vi "Analysis.Result Summaries, Calculate Yield Metrics.vi"(5 "Total Cnt":i32, 6 "Retries":i32[](array[numeric]), 7 "Pass Cnt":i32, 8 "LP Fail":i32, 9 "LP Pass":i32, 10 "FP Fail":i32, 11 "FP Pass":i32) -> (3 "Metrics Table":string[][](table))   [LabVIEW 2024]
uses:
  Analysis.Yield Metrics.ctl
panel:
  out "Yield Metrics":T1 {"Retest"."Retested SN %" format="%.2f"; "Last Pass"."Yield%" format="%.2f"; "First Pass"."Yield%" format="%.2f"; "Overall"."Churn %" format="%.2f"; "Overall"."Yield%" format="%.2f"}
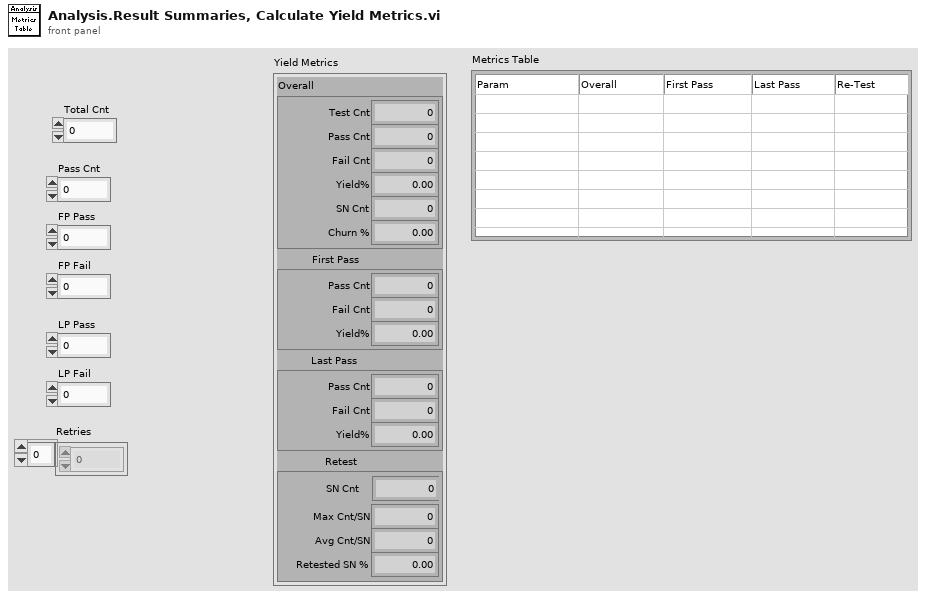
[diagram p1: front panel]
types:
  T1 = typedef "Analysis.Yield Metrics.ctl" = cluster{"Overall":cluster{"Pass Cnt":i32, "Fail Cnt":i32, "Yield%":dbl, "Test Cnt":i32, "SN Cnt":i32, "Churn %":dbl}, "First Pass":cluster{"Pass Cnt":i32, "Fail Cnt":i32, "Yield%":dbl}, "Last Pass":cluster{"Pass Cnt":i32, "Fail Cnt":i32, "Yield%":dbl}, "Retest":cluster{"Max Cnt/SN":i32, "Avg Cnt/SN":i32, "Retested SN %":dbl, "SN Cnt":i32}}
  T2 = cluster{"Pass Cnt":i32, "Fail Cnt":i32, "Yield%":dbl, "Test Cnt":i32, "SN Cnt":i32, "Churn %":dbl}
  T3 = cluster{"Max Cnt/SN":i32, "Avg Cnt/SN":i32, "Retested SN %":dbl, "SN Cnt":i32}
  T4 = cluster{"Pass Cnt":i32, "Fail Cnt":i32, "Yield%":dbl}
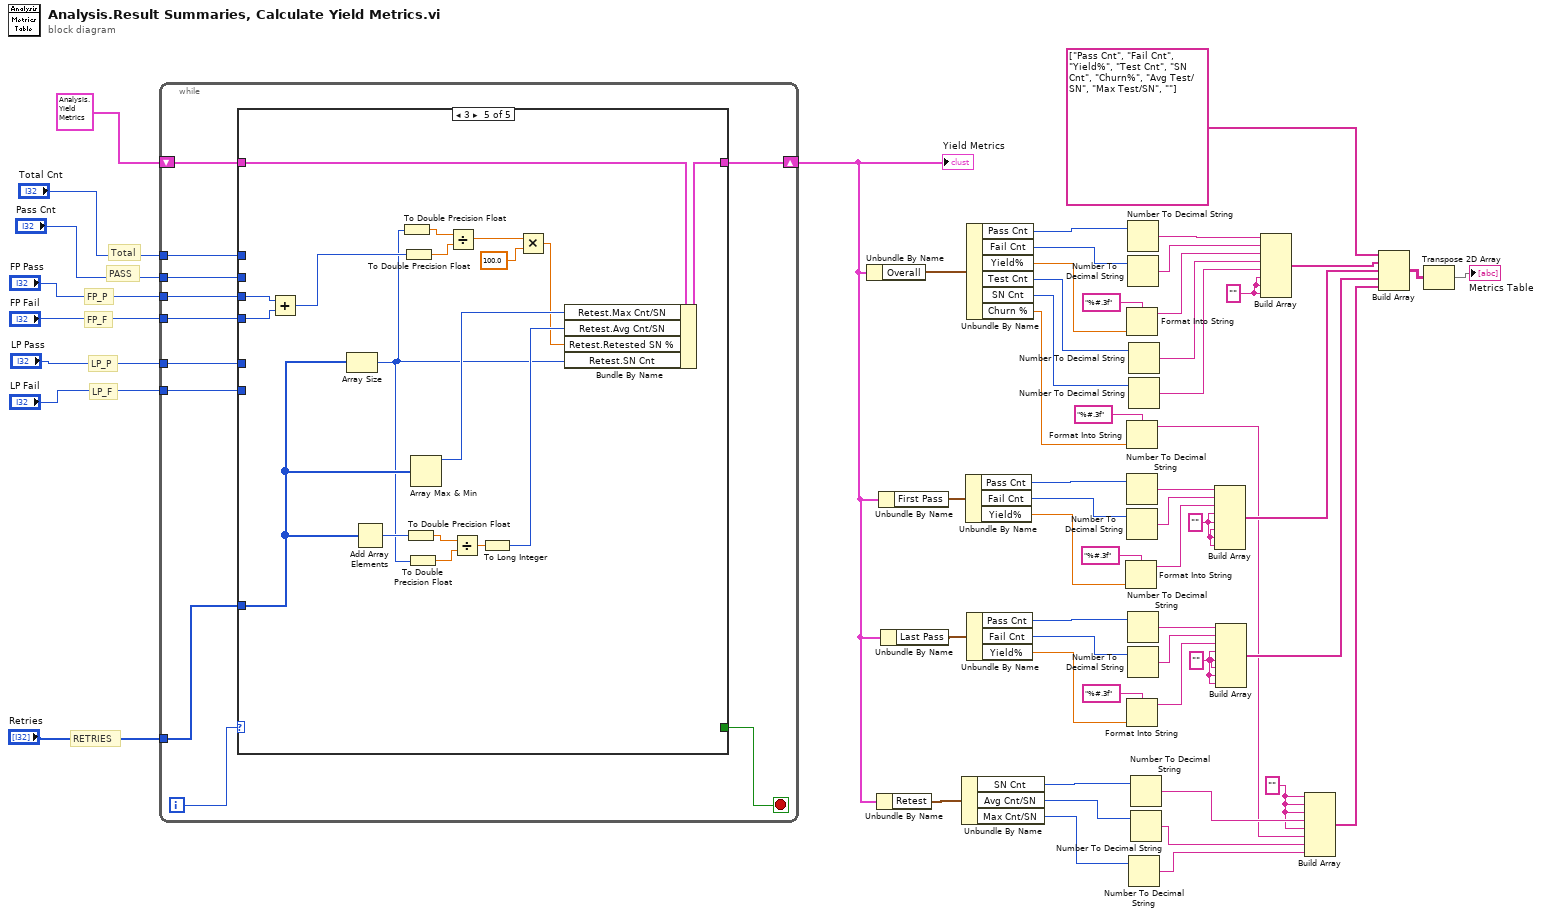
[diagram p0: block diagram]
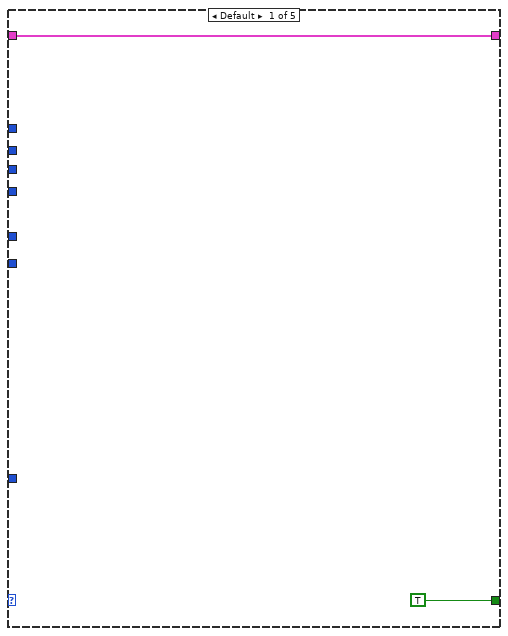
[diagram p2: hidden frame]
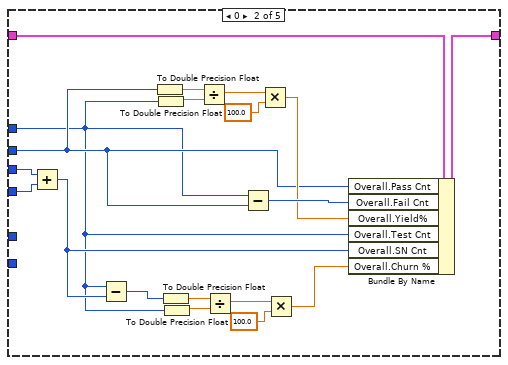
[diagram p3: hidden frame]
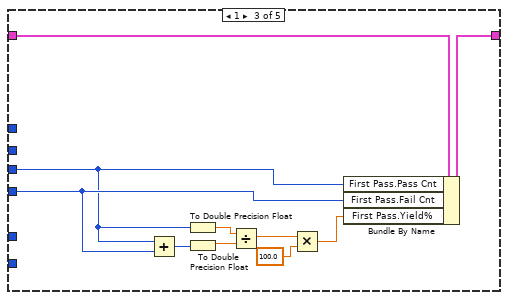
[diagram p4: hidden frame]
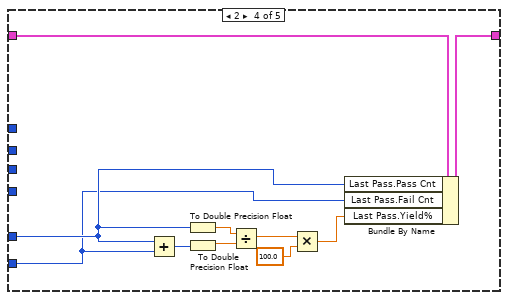
[diagram p5: hidden frame]
diagram:
  w9 = ""
  w17 = ""
  w18 = ""
  w19 = ""
  # "RETRIES"
  # "LP_F"
  # "LP_P"
  # "FP_F"
  # "FP_P"
  # "PASS"
  # "Total"
  n1 = while {
    tunnel: "Total Cnt" -> [w64]
    tunnel: "Pass Cnt" -> [w63]
    tunnel: "FP Pass" -> [w65]
    tunnel: "FP Fail" -> [w60]
    tunnel: "LP Pass" -> [w62]
    tunnel: "LP Fail" -> [w61]
    tunnel: "Retries" -> [w66]
    shift-right: [w68] -> w21
    shift-left: T1 {"Overall"={"Pass Cnt"=0, "Fail Cnt"=0, "Yield%"=0.0, "Test Cnt"=0, "SN Cnt"=0, "Churn %"=0.0}, "First Pass"={"Pass Cnt"=0, "Fail Cnt"=0, "Yield%"=0.0}, "Last Pass"={"Pass Cnt"=0, "Fail Cnt"=0, "Yield%"=0.0}, "Retest"={"Max Cnt/SN"=0, "Avg Cnt/SN"=0, "Retested SN %"=0.0, "SN Cnt"=0}} ("Yield Metrics") -> [w69]
    i -> [w67]
    stop <- w59 stop-if-true
    n2 = case shown="3" w67 {
      tunnel: w69 -> [w71 w89 w99 w109 w127]
      tunnel: [w71 w90 w100 w110 w128] -> w68
      tunnel: w66 -> [_ _ _ _ w121]
      tunnel: w65 -> [_ w85 w91 _ w117]
      tunnel: w64 -> [_ w72 _ _ _]
      tunnel: w63 -> [_ w73 _ _ _]
      tunnel: w62 -> [_ _ _ w102 _]
      tunnel: w61 -> [_ _ _ w101 _]
      tunnel: w60 -> [_ w84 w92 _ w116]
      tunnel: [TRUE _ _ _ _] -> w59
      frame Default {
      }
      frame 0 {
        n3 = Add(x=w85, y=w84) -> (x+y=w74:i32)
        n4 = Subtract(x=w72, y=w74) -> (x-y=w81:i32)
        n5 = To Double Precision Float(number=w73) -> (double precision float=w79:dbl)
        n6 = To Double Precision Float(number=w72) -> (double precision float=w78:dbl)
        n7 = To Double Precision Float(number=w81) -> (double precision float=w82:dbl)
        n8 = To Double Precision Float(number=w72) -> (double precision float=w83:dbl)
        n9 = Divide(x=w79, y=w78) -> (x/y=w76:dbl)
        n10 = Divide(x=w82, y=w83) -> (x/y=w87:dbl)
        n11 = Subtract(x=w72, y=w73) -> (x-y=w88:i32)
        n12 = Multiply(x=w76, y=100.0) -> (x*y=w75:dbl)
        n13 = Multiply(x=w87, y=100.0) -> (x*y=w80:dbl)
        n14 = Bundle By Name(cluster=w89, "Overall.Pass Cnt"=w73, "Overall.Fail Cnt"=w88, "Overall.Yield%"=w75, "Overall.Test Cnt"=w72, "Overall.SN Cnt"=w74, "Overall.Churn %"=w80) -> (w90:T1)
      }
      frame 1 {
        n15 = Add(x=w91, y=w92) -> (x+y=w93:i32)
        n16 = To Double Precision Float(number=w91) -> (double precision float=w94:dbl)
        n17 = To Double Precision Float(number=w93) -> (double precision float=w97:dbl)
        n18 = Divide(x=w94, y=w97) -> (x/y=w98:dbl)
        n19 = Multiply(x=w98, y=100.0) -> (x*y=w95:dbl)
        n20 = Bundle By Name(cluster=w99, "First Pass.Pass Cnt"=w91, "First Pass.Fail Cnt"=w92, "First Pass.Yield%"=w95) -> (w100:T1)
      }
      frame 2 {
        n21 = Add(x=w102, y=w101) -> (x+y=w103:i32)
        n22 = To Double Precision Float(number=w102) -> (double precision float=w104:dbl)
        n23 = To Double Precision Float(number=w103) -> (double precision float=w107:dbl)
        n24 = Divide(x=w104, y=w107) -> (x/y=w108:dbl)
        n25 = Multiply(x=w108, y=100.0) -> (x*y=w105:dbl)
        n26 = Bundle By Name(cluster=w109, "Last Pass.Pass Cnt"=w102, "Last Pass.Fail Cnt"=w101, "Last Pass.Yield%"=w105) -> (w110:T1)
      }
      frame 3 {
        n27 = Add(x=w117, y=w116) -> (x+y=w115:i32)
        n28 = Array Size(array=w121) -> (size(s)=w114:i32)
        n29 = Add Array Elements(numeric array=w121) -> (sum=w126:i32)
        n30 = To Double Precision Float(number=w114) -> (double precision float=w118:dbl)
        n31 = To Double Precision Float(number=w115) -> (double precision float=w119:dbl)
        n32 = To Double Precision Float(number=w126) -> (double precision float=w125:dbl)
        n33 = To Double Precision Float(number=w114) -> (double precision float=w124:dbl)
        n34 = Array Max & Min(array=w121) -> (max value=w120:i32)  [unwired: 3 out]
        n35 = Divide(x=w118, y=w119) -> (x/y=w112:dbl)
        n36 = Divide(x=w125, y=w124) -> (x/y=w123:dbl)
        n37 = To Long Integer(number=w123) -> (32bit integer=w122:i32)
        n38 = Multiply(x=w112, y=100.0) -> (x*y=w111:dbl)
        n39 = Bundle By Name(cluster=w127, "Retest.Max Cnt/SN"=w120, "Retest.Avg Cnt/SN"=w122, "Retest.Retested SN %"=w111, "Retest.SN Cnt"=w114) -> (w128:T1)
      }
    }
  }
  "Yield Metrics" <- w21
  n40 = Unbundle By Name(w21) -> ("Overall"=w57:T2)
  n41 = Unbundle By Name(w21) -> ("Retest"=w33:T3)
  n42 = Unbundle By Name(w21) -> ("First Pass"=w34:T4)
  n43 = Unbundle By Name(w21) -> ("Last Pass"=w29:T4)
  n44 = Unbundle By Name(w33) -> ("SN Cnt"=w32:i32, "Avg Cnt/SN"=w31:i32, "Max Cnt/SN"=w30:i32)
  n45 = Unbundle By Name(w34) -> ("Pass Cnt"=w35:i32, "Fail Cnt"=w36:i32, "Yield%"=w38:dbl)
  n46 = Unbundle By Name(w57) -> ("Pass Cnt"=w56:i32, "Fail Cnt"=w55:i32, "Yield%"=w52:dbl, "Test Cnt"=w51:i32, "SN Cnt"=w50:i32, "Churn %"=w49:dbl)
  n47 = Unbundle By Name(w29) -> ("Pass Cnt"=w28:i32, "Fail Cnt"=w27:i32, "Yield%"=w25:dbl)
  n48 = Format Into String(format string="%#.3f", w38) -> (resulting string=w41:string)  [unwired: 2 in, 1 out]
  n49 = Format Into String(format string="%#.3f", w52) -> (resulting string=w46:string)  [unwired: 2 in, 1 out]
  n50 = Format Into String(format string="%#.3f", w49) -> (resulting string=w8:string)  [unwired: 2 in, 1 out]
  n51 = Number To Decimal String(number=w35) -> (decimal integer string=w39:string)  [unwired: 1 in]
  n52 = Number To Decimal String(number=w36) -> (decimal integer string=w40:string)  [unwired: 1 in]
  n53 = Format Into String(format string="%#.3f", w25) -> (resulting string=w22:string)  [unwired: 2 in, 1 out]
  n54 = Number To Decimal String(number=w56) -> (decimal integer string=w48:string)  [unwired: 1 in]
  n55 = Number To Decimal String(number=w55) -> (decimal integer string=w47:string)  [unwired: 1 in]
  n56 = Number To Decimal String(number=w28) -> (decimal integer string=w24:string)  [unwired: 1 in]
  n57 = Number To Decimal String(number=w27) -> (decimal integer string=w23:string)  [unwired: 1 in]
  n58 = Number To Decimal String(number=w51) -> (decimal integer string=w45:string)  [unwired: 1 in]
  n59 = Number To Decimal String(number=w50) -> (decimal integer string=w44:string)  [unwired: 1 in]
  n60 = Number To Decimal String(number=w30) -> (decimal integer string=w15:string)  [unwired: 1 in]
  n61 = Number To Decimal String(number=w32) -> (decimal integer string=w20:string)  [unwired: 1 in]
  n62 = Number To Decimal String(number=w31) -> (decimal integer string=w16:string)  [unwired: 1 in]
  n63 = Build Array(w39, w40, w41, w19, w19, w19, w19, w19) -> (w14:string[])
  n64 = Build Array(w24, w23, w22, w18, w18, w18, w18, w18) -> (w13:string[])
  n65 = Build Array(w48, w47, w46, w45, w44, w9, w9, w9) -> (w42:string[])
  n66 = Build Array(w17, w17, w17, w20, w17, w8, w16, w15) -> (w12:string[])
  n67 = Build Array(string[] ["Pass Cnt", "Fail Cnt", "Yield%", "Test Cnt", "SN Cnt", "Churn%", "Avg Test/SN", "Max Test/SN", ""] ("subarray"), w42, w14, w13, w12) -> (w11:string[][])
  n68 = Transpose 2D Array(2D array=w11) -> (transposed array=→"Metrics Table":string[][])
